vi "NF WF1973_74 TRAC Inf.vi"(7 "Memory No.(0)":i32 min=0 max=128 step=1, 8 "error in (no error)":errorcluster caption="Error IN", 11 "VISAsession":refnum<visa-resource-name>) -> (0 "error out":errorcluster caption="Error OUT", 2 "Information":string, 3 "CopyVISAsession":refnum<visa-resource-name>)   [LabVIEW 2010]
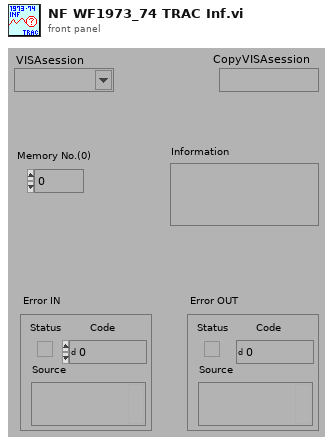
[diagram p1: front panel]
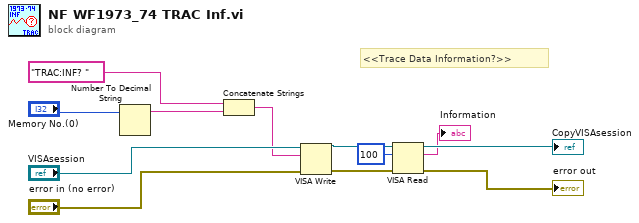
[diagram p0: block diagram]
diagram:
  # "<<Trace Data Information?>>"
  n1 = Number To Decimal String(number="Memory No.(0)") -> (decimal integer string=w8:string)  [unwired: 1 in]
  n2 = Concatenate Strings("TRAC:INF? ", w8) -> (w7:string)
  n3 = VISA Write(VISA resource name="VISAsession", write buffer=w7, error in (no error)="error in (no error)") -> (VISA resource name out=w4:refnum<visa-resource-name>, error out=w5:errorcluster)  [unwired: 1 out]
  n4 = VISA Read(VISA resource name=w4, byte count=u32 100 ("バイトカウント（0）"), error in (no error)=w5) -> (VISA resource name out=→"CopyVISAsession":refnum<visa-resource-name>, read buffer=→"Information":string, error out=→"error out":errorcluster)  [unwired: 1 out]
